vi "CreateNewProj.vi"() -> ()   [LabVIEW 2026]
panel:
  out "error out":errorcluster
  in  "error in (no error)":errorcluster
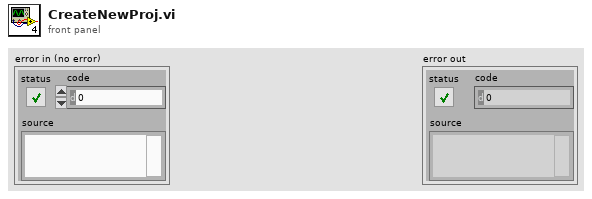
[diagram p1: front panel]
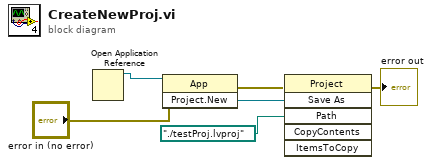
[diagram p0: block diagram]
diagram:
  n1 = Open Application Reference() -> (3:w6:refnum<vi>)  [unwired: 4 in, 1 out]
  n2 = invoke class="App" method="Project.New"(reference=w6, error in="error in (no error)") -> (error out=w2:errorcluster, "Project:New"=w5:refnum<vi>)  [unwired: 1 in, 1 out]
  n3 = invoke class="Project" method="Save As"(reference=w5, error in=w2, "Path"=path "./testProj.lvproj") -> (error out=→"error out":errorcluster)  [unwired: 3 in, 5 out]
